vi "Real Sine-waves from Complex.vi"(8 "Error In":errorcluster, 9 "Complex Waveforms In":waveform(cdb)[](array[waveform])) -> (0 "Error Out":errorcluster, 1 "Real Waveforms Out":waveform(dbl)[](array[waveform]))   [LabVIEW 2019]
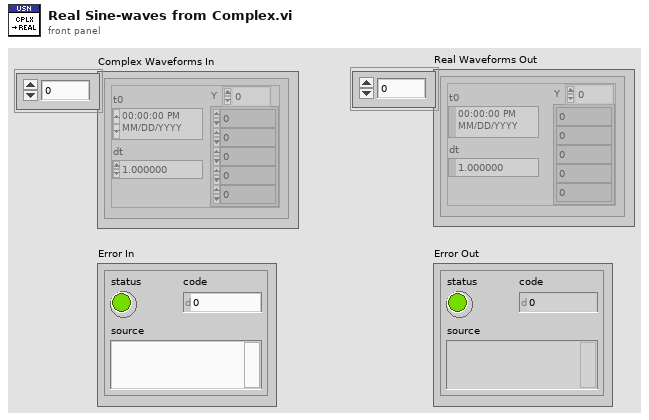
[diagram p1: front panel]
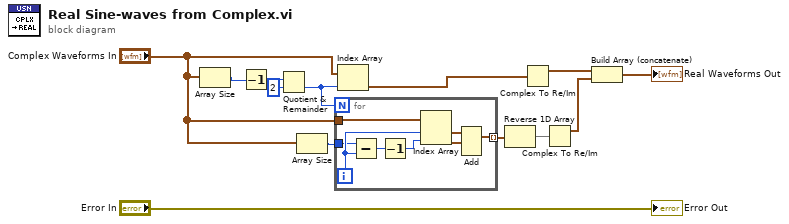
[diagram p0: block diagram]
diagram:
  n1 = Array Size(array="Complex Waveforms In") -> (size(s)=w4:i32)
  n2 = Decrement(x=w4) -> (x-1=w3:i32)
  n3 = Quotient & Remainder(x=w3, y=2) -> (floor(x/y)=w1:i32)  [unwired: 1 out]
  n4 = Array Size(array="Complex Waveforms In") -> (size(s)=w13:i32)
  n5 = for {
    N: w1 -> [_]
    tunnel: "Complex Waveforms In" -> [w21]
    tunnel: [w16] -> w12 mode=indexing
    tunnel: w13 -> [w15]
    i -> [w20]
    n6 = Subtract(x=w15, y=w20) -> (x-y=w19:i32)
    n7 = Decrement(x=w19) -> (x-1=w14:i32)
    n8 = Index Array(array=w21, index #1=w20, index #2=w14) -> (element #1=w18:waveform(cdb), element #2=w17:waveform(cdb))
    n9 = Add(1:w17, 2:w18) -> (0:w16:waveform(cdb))  [unwired: 1 in, 1 out]
  }
  n10 = Index Array(array="Complex Waveforms In", index=w1) -> (element=w8:waveform(cdb))
  n11 = Reverse 1D Array(array=w12) -> (reversed array=w9:waveform(cdb)[])
  n12 = Complex To Re/Im(x + iy=w8) -> (x=w7:waveform(dbl))  [unwired: 1 out]
  n13 = Complex To Re/Im(x + iy=w9) -> (x=w6:waveform(dbl)[])  [unwired: 1 out]
  n14 = Build Array (concatenate)(w7, w6) -> (→"Real Waveforms Out":waveform(dbl)[])
  "Error Out" <- "Error In"
